vi "MRaySelectShooterFile.vi"(10 "Shooter File":dbl) -> ()   [LabVIEW 2011]
uses:
  <vilib>/Rock Robotics/WPI/DriverStation/DriverStationLCD/WPI_DriverStationLCDLCDLine.ctl
  2012 Robot Code 2-23-12 Comp Bot/Robot Global Data.vi
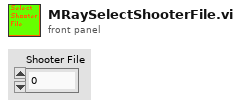
[diagram p1: front panel]
types:
  T1 = typedef "WPI_DriverStationLCDLCDLine.ctl" = enum16{"Main - Line 1", "User - Line 2", "User - Line 3", "User - Line 4", "User - Line 5", "User - Line 6"}
  T2 = enum16{"False", "FalseToTrue", "True", "TrueToFalse"}
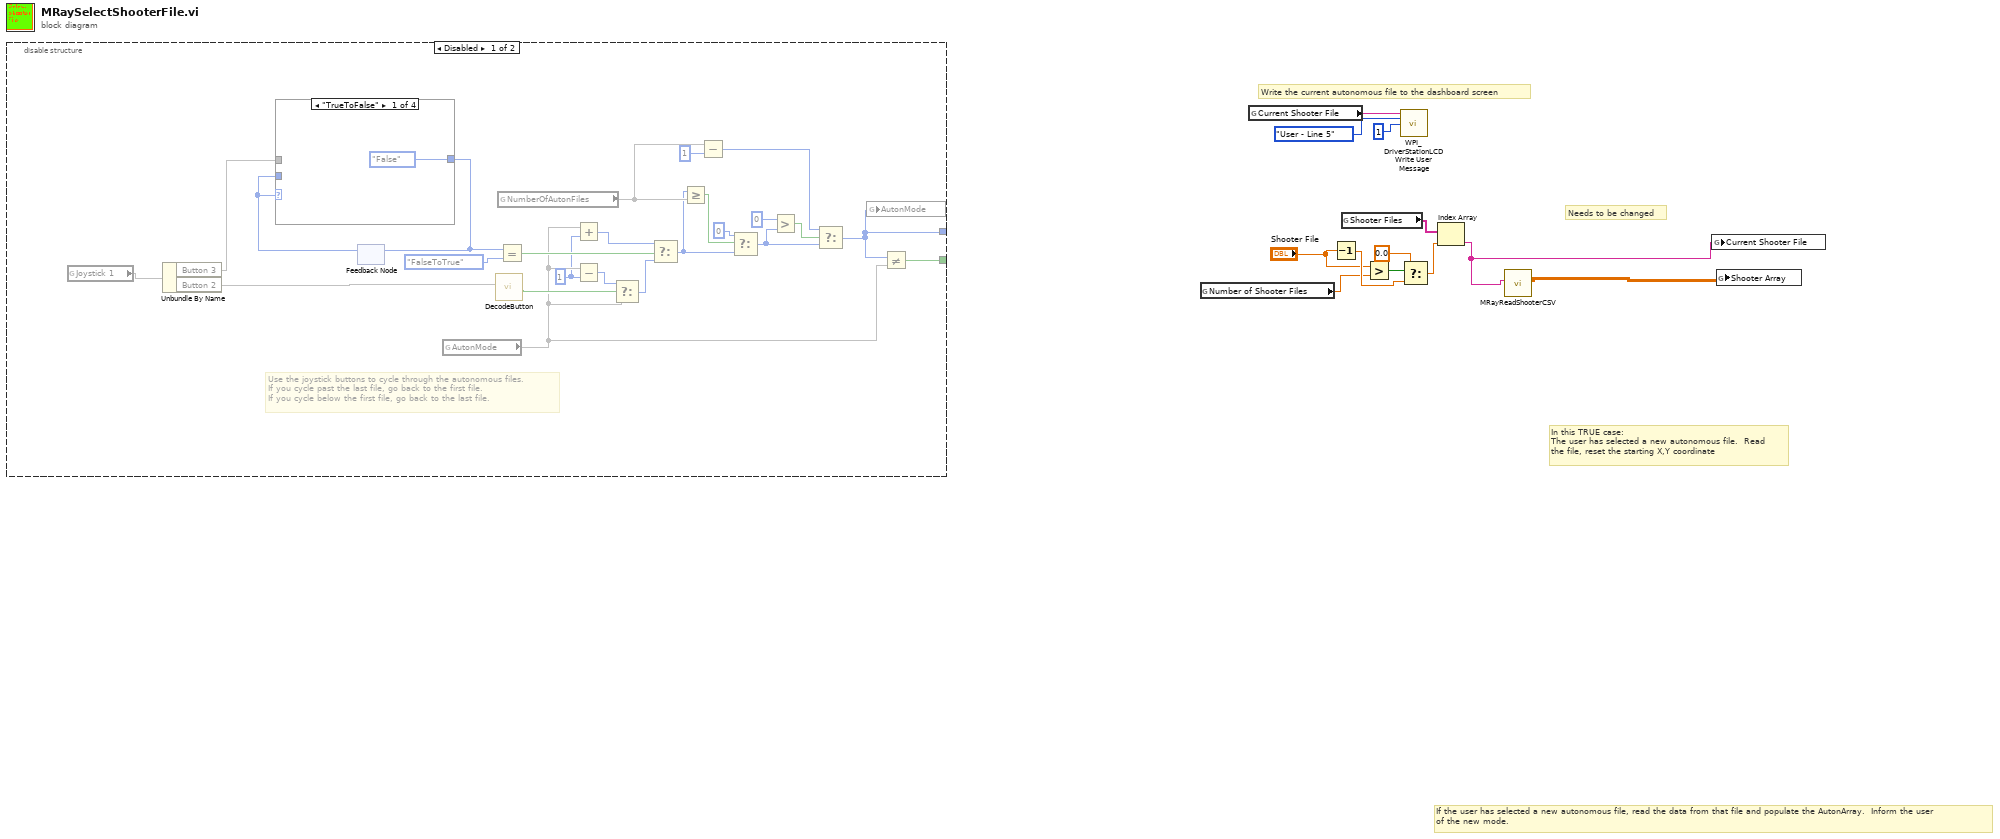
[diagram p0: block diagram]
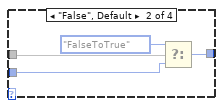
[diagram p2: hidden frame]
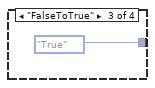
[diagram p3: hidden frame]
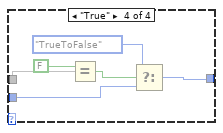
[diagram p4: hidden frame]
diagram:
  # "Needs to be changed"
  # "In this TRUE case:\nThe user has selected a new autonomous file.  Read\nthe file, reset the starting X,Y coordinate"
  # "Write the current autonomous file to the dashboard screen"
  # "If the user has selected a new autonomous file, read the data from that file and populate the AutonArray.  Inform the user\nof the new mode."
  n1 = disable-structure shown="Disabled" {
    disable-tunnel: [w36 _] -> _
    disable-tunnel: [w26 _] -> _
    frame Disabled {
      w17 = i16 1 ("y")
      # "Use the joystick buttons to cycle through the autonomous files.\nIf you cycle past the last file, go back to the first file.\nIf you cycle below the first file, go back to the last file."
      n2 = global read "Robot Global Data.vi" "Joystick 1"() -> (w13)
      n3 = Unbundle By Name(w13) -> ("Button 3"=w24, "Button 2"=w14)
      n4 = feedback #1() -> (w21:T2)  [unwired: 1 out]
      n5 = case shown="\"TrueToFalse\"" w21 {
        tunnel: w24 -> [_ w41 _ w47]
        tunnel: [T2."False" ("f") w39 T2."True" ("y") w48] -> w22
        tunnel: w21 -> [_ w38 _ w44]
        frame "TrueToFalse" {
        }
        frame "False", Default {
          n6 = Select(t=T2."FalseToTrue", s=w41, f=w38) -> (s? t:f=w39:T2)
        }
        frame "FalseToTrue" {
        }
        frame "True" {
          n7 = Equal?(x=FALSE, y=w47) -> (x = y?=w45:bool)
          n8 = Select(t=T2."TrueToFalse", s=w45, f=w44) -> (s? t:f=w48:T2)
        }
      }
      n9 = feedback-in #1(w22) -> ()
      n10 = global read "Robot Global Data.vi" "AutonMode"() -> (w19)
      n11 = call "DecodeButton.vi"("Button"=w14) -> ("False to True"=w20:bool)  [unwired: 10 out]
      n12 = global read "Robot Global Data.vi" "NumberOfAutonFiles"() -> (w33)
      n13 = Equal?(x=w22, y=T2."FalseToTrue") -> (x = y?=w25:bool)
      n14 = Add(x=w19, y=w17) -> (x+y=w18:i16)
      n15 = Subtract(x=w19, y=w17) -> (x-y=w15:i16)
      n16 = Select(t=w15, s=w20, f=w19) -> (s? t:f=w16:i16)
      n17 = Select(t=w18, s=w25, f=w16) -> (s? t:f=w27:i16)
      n18 = Greater Or Equal?(x=w27, y=w33) -> (x >= y?=w28:bool)
      n19 = Subtract(x=w33, y=i16 1) -> (x-y=w35:i16)
      n20 = Select(t=i16 0, s=w28, f=w27) -> (s? t:f=w30:i16)
      n21 = Greater?(x=i16 0, y=w30) -> (0:w32:bool)
      n22 = Select(t=w35, s=w32, f=w30) -> (s? t:f=w36:i16)
      n23 = global write "Robot Global Data.vi" "AutonMode"(w36) -> ()
      n24 = Not Equal?(x=w36, y=w19) -> (x != y?=w26:bool)
    }
    frame Enabled {
    }
  }
  n25 = global read "Robot Global Data.vi" "Number of Shooter Files"() -> (w2:dbl)
  n26 = global read "Robot Global Data.vi" "Current Shooter File"() -> (w10:string)
  n27 = Decrement(x="Shooter File") -> (x-1=w4:dbl)
  n28 = global read "Robot Global Data.vi" "Shooter Files"() -> (w9:string[])
  n29 = Greater?(x="Shooter File", y=w2) -> (0:w6:bool)
  n30 = call <vilib>:"WPI_DriverStationLCDWrite User Message.vi"("line text"=w10, "line"=WPI_DriverStationLCDLCDLine."User - Line 5", "starting column"=i8 1) -> ()  [unwired: 2 in, 11 out]
  n31 = Select(t=0.0, s=w6, f=w4) -> (s? t:f=w1:dbl)
  n32 = Index Array(array=w9, index=w1) -> (element=w8:string)
  n33 = call "MRayReadShooterCSV.vi"("ShooterFile"=w8) -> ("ShooterArray"=w7:dbl[][])  [unwired: 10 in]
  n34 = global write "Robot Global Data.vi" "Current Shooter File"(w8) -> ()
  n35 = global write "Robot Global Data.vi" "Shooter Array"(w7) -> ()
